vi "calDecimateTS.vi"(10 "660 Data":dbl[](array[numeric]), 11 "532 Data":dbl[](array[numeric])) -> (2 "Decimated 660":dbl[](array[numeric]), 3 "Decimated 532":dbl[](array[numeric]))   [LabVIEW 2011]
uses:
  <vilib>/Analysis/NI_AALBase.lvlib
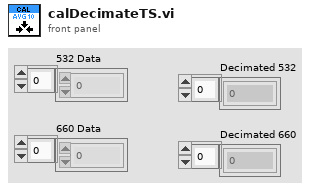
[diagram p1: front panel]
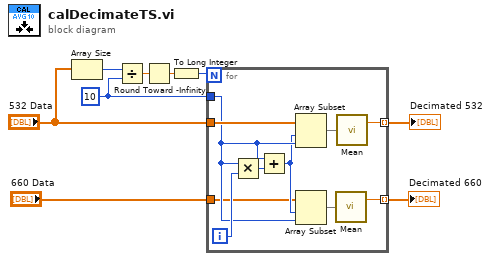
[diagram p0: block diagram]
diagram:
  w7 = 10 ("y")
  n1 = Array Size(array="532 Data") -> (size(s)=w2:i32)
  n2 = Divide(x=w2, y=w7) -> (x/y=w6:dbl)
  n3 = Round Toward -Infinity(1:w6) -> (0:w4:dbl)
  n4 = To Long Integer(number=w4) -> (32bit integer=w5:i32)
  n5 = for {
    N: w5 -> [_]
    tunnel: "532 Data" -> [w19]
    tunnel: [w18] -> w9 mode=indexing
    tunnel: w7 -> [w14]
    tunnel: [w15] -> w8 mode=indexing
    tunnel: "660 Data" -> [w11]
    i -> [w17]
    n6 = Multiply(x=w14, y=w17) -> (x*y=w16:i32)
    n7 = Add(x=w14, y=w16) -> (x+y=w13:i32)
    n8 = Array Subset(array=w19, index=w13, length=w14) -> (w12:dbl[])
    n9 = Array Subset(array=w11, index=w13, length=w14) -> (w10:dbl[])
    n10 = call <vilib>:"Mean.vi"("X"=w10) -> ("mean"=w15:dbl)  [unwired: 1 out]
    n11 = call <vilib>:"Mean.vi"("X"=w12) -> ("mean"=w18:dbl)  [unwired: 1 out]
  }
  "Decimated 532" <- w9
  "Decimated 660" <- w8
